vi "Stop Core.vi"(10 "final error code":i32, 11 "Stage in":refnum<class "Stage.lvclass">) -> (3 "Stage out":refnum<class "Stage.lvclass">)   [LabVIEW 2018, in "Stage Actor.lvlib" / "Stage.lvclass"]
doc: "In override VIs of Stop Core.vi, an actor should invoke any code needed to stop all the parallel processes that it created during its run. This includes any nested actors that it created and any other asynchronously running VIs, such as a Time-Delayed Message. It may also include all parallel loops in its Actor Core, although it is acceptable to stop those using a local signal on the Actor Core block diagram that is raised after the Call Parent Node finishes. \n\nThe <b>final error code</b> input tells the actor what error was set when this actor quit. Zero means there was no error. You can use this to decide whether this should be treated as a Normal Stop or an Emergency Stop for the purposes of signaling other actors. In general, any non-zero value should be treated as an Emergency Stop, though a given actor is free to choose other policies. Note that the particular error code 1608 indicates that this actor was itself stopped by an Emergency Stop and should pass that along."
uses:
  Stage.lvclass
  Stage.lvclass/Stage.ctl
  <vilib>/MGI/Panel Manager/Panel Actor/Panel Actor/Panel Actor.lvclass
  <instrlib>/Zaber A Series/Zaber A Series.lvlib
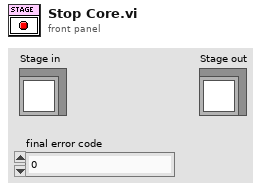
[diagram p1: front panel]
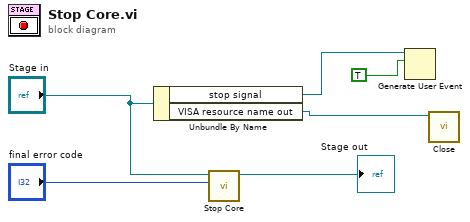
[diagram p0: block diagram]
diagram:
  n1 = Unbundle By Name("Stage in") -> ("stop signal"=w3:refnum<user-event>, "VISA resource name out"=w1:refnum<visa-resource-name>)
  n2 = call-parent "Stop Core.vi"("final error code"="final error code", "Monitored Actor in"="Stage in") -> ("Monitored Actor out"=→"Stage out":refnum<class "Stage.lvclass">)  [unwired: 9 in]
  n3 = Generate User Event(user event=w3, event data cluster=TRUE) -> ()  [unwired: 2 in, 2 out]
  n4 = call <instrlib>:"Close.vi"("VISA resource name"=w1) -> ()  [unwired: 10 in, 1 out]
